vi "Depth and Stainless Correction Pop Up 2016.vi"(6 "New Number\n of Stainless\n(Count)":i32, 7 "Input \nCorrected \nDepth (Feet)":sgl format="%.2f") -> (0 "Array":u16[](array[numeric]), 1 "Record IK Reason 2":bool, 2 "Feet of\nStainless to be\nUsed (Count)":i32, 3 "Depth to \nbe Used \n(Feet)":sgl format="%.2f", 4 "IK Log Note 2":string, 5 "End of Hole 2":u16(ring) items=["ROP Dropped below threshold", "Sudden hard refusal", "Reached target depth", "Broken down hole equipment", "Other"])   [LabVIEW 2016]
doc: "This vi allows the clinician to input the starting flexion. It used in order to derive a flexion correction."
panel:
  in  "End of Hole":u16(ring)=4 items=["ROP Dropped below threshold", "Sudden hard refusal", "Reached target depth", "Broken down hole equipment", "Other"]
  in  "IK Log Note":string
  out "loop counter":i32
  in  "Select Entry \nfor IK Log":u16(ring)=3 items=["IK Increase", "IK stayed the Same", "IK decreased", "Other"]
  in  "Record IK Reason":bool
  out "Original \nUncorrected \nDepth (Feet)":sgl format="%.2f"
  out "Original Feet\n of Stainless\n(Count)":i32
  in  "stop":bool
  in  "Increment Stainless":bool
  in  "Stainless OK As Is":bool
  in  "Correct Stainless":bool
  in  "Depth OK As Is":bool
  in  "Correct Depth":bool
  # "Please Choose \nto Correct Depth\nor to Leave As Is"
  # "Please Choose \nto Correct, Increment, or to \nLeave Feet of Stainless as is"
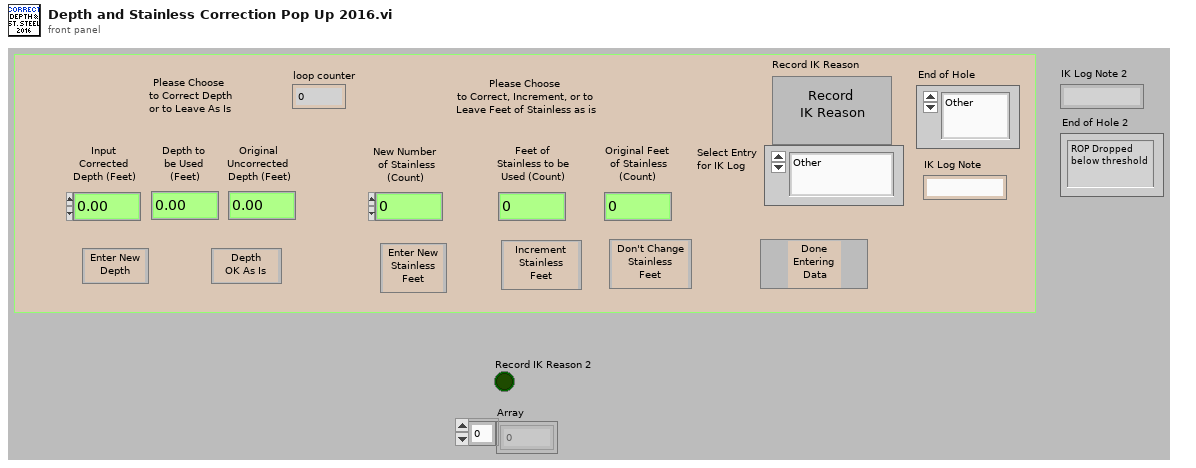
[diagram p1: front panel]
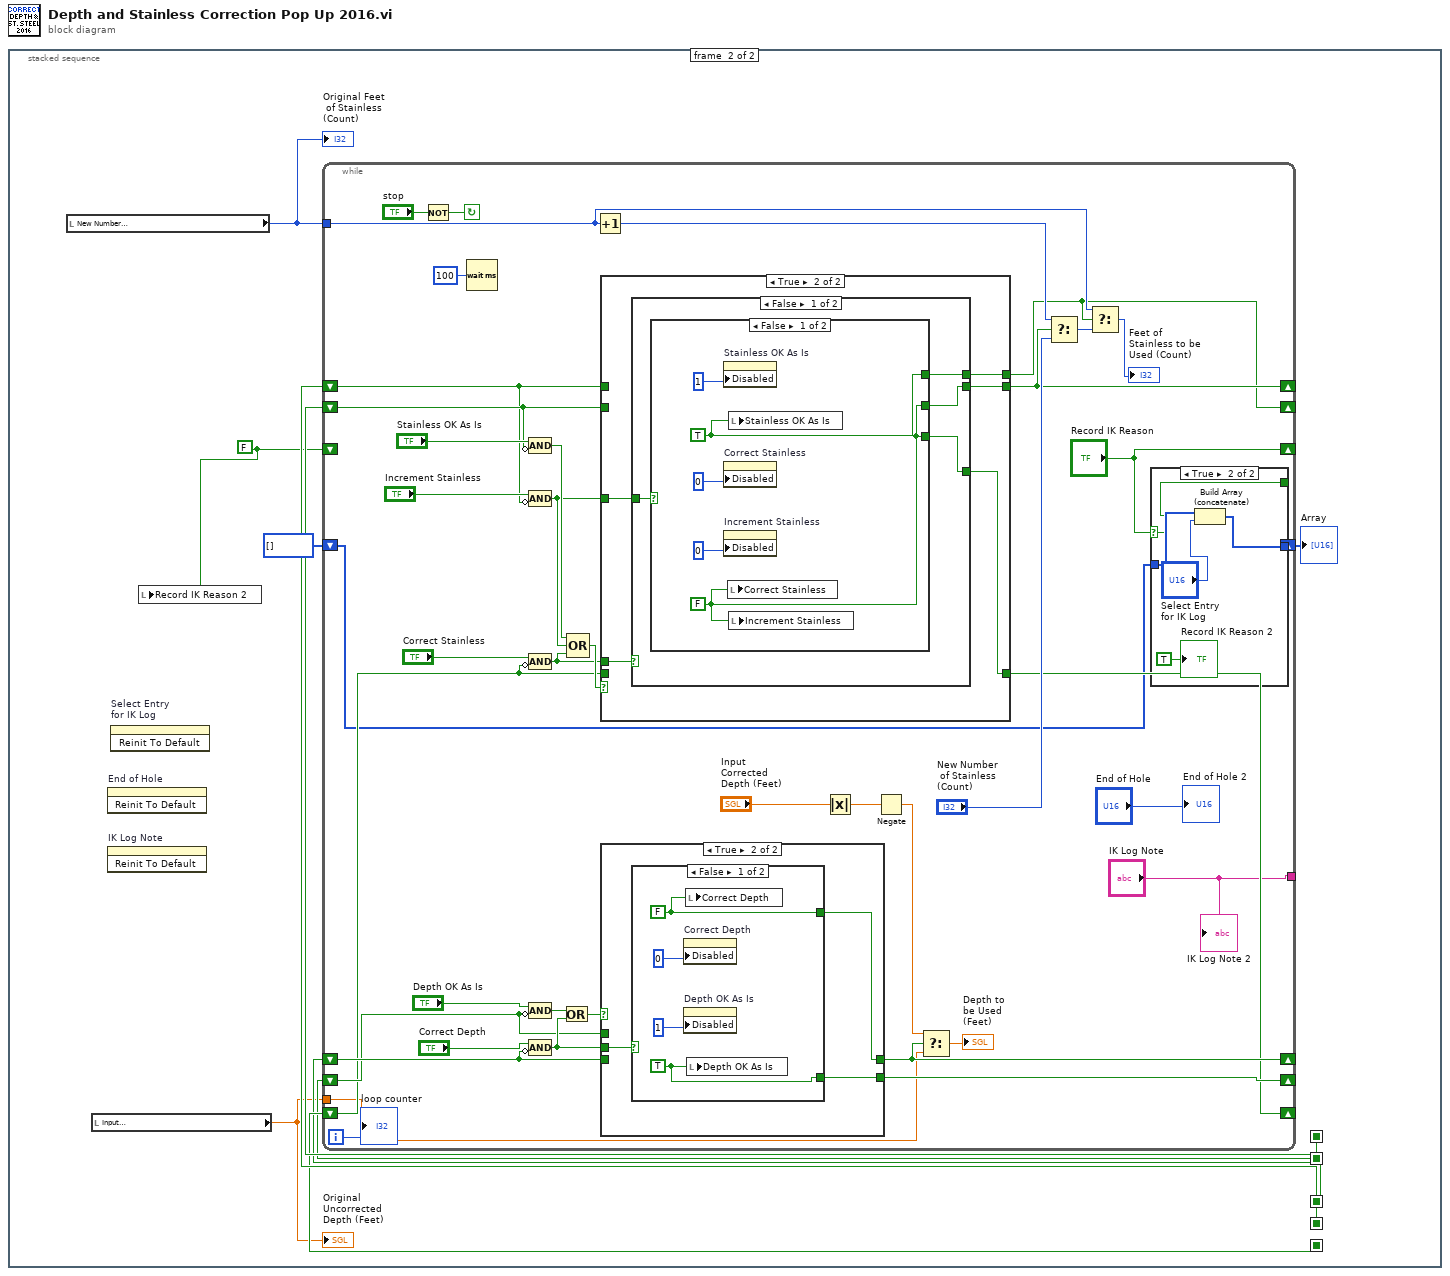
[diagram p0: block diagram]
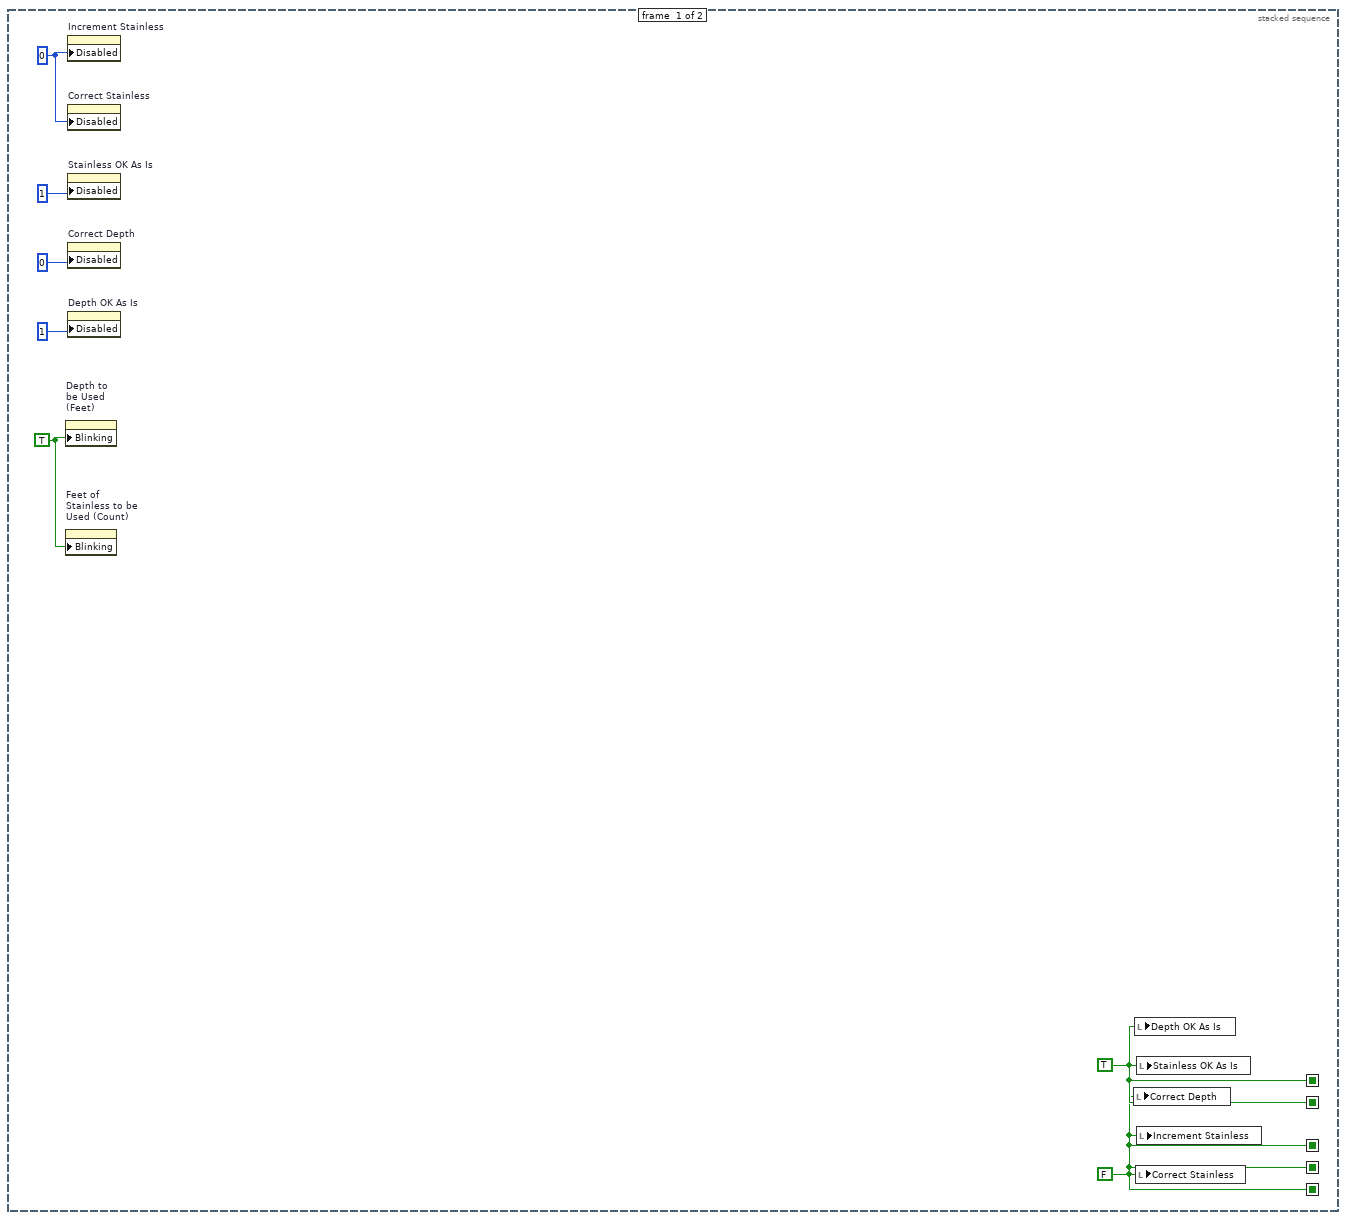
[diagram p2: hidden frame]
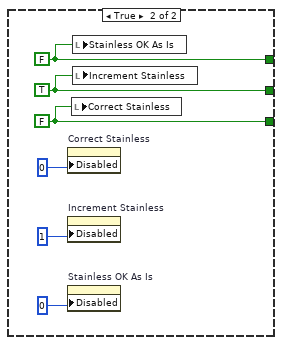
[diagram p5: hidden frame]
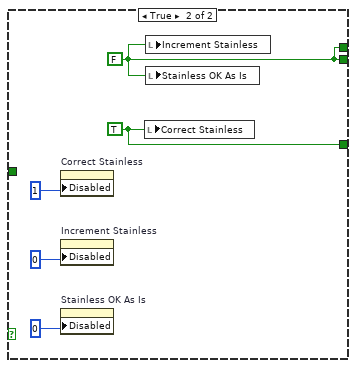
[diagram p6: hidden frame]
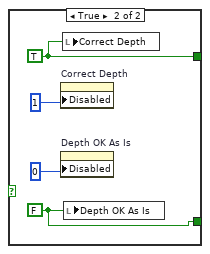
[diagram p8: hidden frame]
diagram:
  n1 = stacked-sequence {
    seq-local: [w6 _] -> [_ w15]
    seq-local: [w6 _] -> [_ w16]
    seq-local: [w7 _] -> [_ w17]
    seq-local: [w6 _] -> [_ w13]
    seq-local: [w7 _] -> [_ w14]
    frame #0 {
      w1 = TRUE
      w2 = 0
      w7 = TRUE
      w6 = FALSE
      n2 = property on="Depth to \nbe Used \n(Feet)" class="DigNum (strict)"("Blinking"=w1) -> ()  [unwired: 2 in, 2 out]
      n3 = property on="Feet of\nStainless to be\nUsed (Count)" class="DigNum (strict)"("Blinking"=w1) -> ()  [unwired: 2 in, 2 out]
      n4 = property on="Increment Stainless" class="Bool (strict)"("Disabled"=w2) -> ()  [unwired: 2 in, 2 out]
      n5 = property on="Correct Stainless" class="Bool (strict)"("Disabled"=w2) -> ()  [unwired: 2 in, 2 out]
      n6 = property on="Stainless OK As Is" class="Bool (strict)"("Disabled"=1) -> ()  [unwired: 2 in, 2 out]
      n7 = property on="Correct Depth" class="Bool (strict)"("Disabled"=0) -> ()  [unwired: 2 in, 2 out]
      n8 = property on="Depth OK As Is" class="Bool (strict)"("Disabled"=1) -> ()  [unwired: 2 in, 2 out]
      n9 = local write "Correct Depth"(w6) -> ()
      n10 = local write "Depth OK As Is"(w7) -> ()
      n11 = local write "Correct Stainless"(w6) -> ()
      n12 = local write "Stainless OK As Is"(w7) -> ()
      n13 = local write "Increment Stainless"(w6) -> ()
    }
    frame #1 {
      w8 = FALSE
      n14 = local read "New Number\n of Stainless\n(Count)"() -> (w12:i32)
      "Original Feet\n of Stainless\n(Count)" <- w12
      n15 = local read "Input \nCorrected \nDepth (Feet)"() -> (w11:sgl)
      "Original \nUncorrected \nDepth (Feet)" <- w11
      n16 = invoke on="End of Hole" class="Ring (strict)" method="Reinit To Default"() -> ()  [unwired: 3 in, 3 out]
      n17 = invoke on="IK Log Note" class="Str" method="Reinit To Default"() -> ()  [unwired: 3 in, 3 out]
      n18 = invoke on="Select Entry \nfor IK Log" class="Ring (strict)" method="Reinit To Default"() -> ()  [unwired: 3 in, 3 out]
      n19 = local write "Record IK Reason 2"(w8) -> ()
      n20 = while {
        tunnel: w11 -> [w29]
        tunnel: w12 -> [w30]
        shift-left: w13 -> [w35]
        shift-right: [w46] -> _
        shift-left: w14 -> [w34]
        shift-right: [w47] -> _
        shift-left: w15 -> [w32]
        shift-right: [w39] -> _
        shift-left: w16 -> [w31]
        shift-right: [w40] -> _
        shift-left: w17 -> [w33]
        shift-right: [w28] -> _
        shift-right: [w24] -> w9
        shift-left: u16[] [] -> [w23]
        shift-right: ["Record IK Reason"] -> _
        shift-left: w8 -> [_]
        tunnel: ["IK Log Note"] -> _
        i -> [w22]
        stop <- w36 continue-if-true
        n21 = Not(x="stop") -> (.not. x?=w36:bool)
        n22 = Wait (ms)(milliseconds to wait=u32 100) -> ()  [unwired: 1 out]
        n23 = Compound Arithmetic op=AND("Stainless OK As Is", invert w33) -> (w42:bool)
        n24 = Compound Arithmetic op=AND("Increment Stainless", invert w31) -> (w37:bool)
        n25 = Compound Arithmetic op=AND("Correct Stainless", invert w32) -> (w38:bool)
        n26 = Compound Arithmetic op=AND("Depth OK As Is", invert w34) -> (w51:bool)
        n27 = Compound Arithmetic op=AND("Correct Depth", invert w35) -> (w49:bool)
        n28 = Or(x=w51, y=w49) -> (x .or. y?=w50:bool)
        n29 = Compound Arithmetic op=OR(w42, w37, w38) -> (w41:bool)
        n30 = Increment(x=w30) -> (x+1=w57:i32)
        n31 = case shown="True" w41 {
          tunnel: [w68 w71] -> w28
          tunnel: [w67 w70] -> w40
          tunnel: [w66 w72] -> w39
          tunnel: w38 -> [_ w73]
          tunnel: w37 -> [_ w69]
          tunnel: w33 -> [w68 _]
          tunnel: w32 -> [w66 _]
          tunnel: w31 -> [w67 _]
          frame False {
          }
          frame True {
            n32 = case shown="False" w73 {
              tunnel: [w74 w93] -> w72
              tunnel: [w76 w92] -> w71
              tunnel: [w75 w92] -> w70
              tunnel: w69 -> [w77 _]
              frame False {
                n33 = case shown="False" w77 {
                  tunnel: [w81 w86] -> w76
                  tunnel: [w82 w87] -> w75
                  tunnel: [w82 w88] -> w74
                  frame False {
                    w81 = TRUE
                    w82 = FALSE
                    n34 = property on="Stainless OK As Is" class="Bool (strict)"("Disabled"=1) -> ()  [unwired: 2 in, 2 out]
                    n35 = property on="Correct Stainless" class="Bool (strict)"("Disabled"=0) -> ()  [unwired: 2 in, 2 out]
                    n36 = property on="Increment Stainless" class="Bool (strict)"("Disabled"=0) -> ()  [unwired: 2 in, 2 out]
                    n37 = local write "Correct Stainless"(w82) -> ()
                    n38 = local write "Stainless OK As Is"(w81) -> ()
                    n39 = local write "Increment Stainless"(w82) -> ()
                  }
                  frame True {
                    w86 = FALSE
                    w87 = TRUE
                    w88 = FALSE
                    n40 = property on="Correct Stainless" class="Bool (strict)"("Disabled"=0) -> ()  [unwired: 2 in, 2 out]
                    n41 = property on="Increment Stainless" class="Bool (strict)"("Disabled"=1) -> ()  [unwired: 2 in, 2 out]
                    n42 = property on="Stainless OK As Is" class="Bool (strict)"("Disabled"=0) -> ()  [unwired: 2 in, 2 out]
                    n43 = local write "Correct Stainless"(w88) -> ()
                    n44 = local write "Stainless OK As Is"(w86) -> ()
                    n45 = local write "Increment Stainless"(w87) -> ()
                  }
                }
              }
              frame True {
                w92 = FALSE
                w93 = TRUE
                n46 = property on="Correct Stainless" class="Bool (strict)"("Disabled"=1) -> ()  [unwired: 2 in, 2 out]
                n47 = property on="Increment Stainless" class="Bool (strict)"("Disabled"=0) -> ()  [unwired: 2 in, 2 out]
                n48 = property on="Stainless OK As Is" class="Bool (strict)"("Disabled"=0) -> ()  [unwired: 2 in, 2 out]
                n49 = local write "Correct Stainless"(w93) -> ()
                n50 = local write "Increment Stainless"(w92) -> ()
                n51 = local write "Stainless OK As Is"(w92) -> ()
              }
            }
          }
        }
        n52 = case shown="True" w50 {
          tunnel: w49 -> [_ w98]
          tunnel: [w95 w96] -> w47
          tunnel: [w94 w97] -> w46
          tunnel: w35 -> [w94 _]
          tunnel: w34 -> [w95 _]
          frame False {
          }
          frame True {
            n53 = case shown="False" w98 {
              tunnel: [w102 w106] -> w97
              tunnel: [w101 w105] -> w96
              frame False {
                w102 = FALSE
                w101 = TRUE
                n54 = property on="Correct Depth" class="Bool (strict)"("Disabled"=0) -> ()  [unwired: 2 in, 2 out]
                n55 = property on="Depth OK As Is" class="Bool (strict)"("Disabled"=1) -> ()  [unwired: 2 in, 2 out]
                n56 = local write "Correct Depth"(w102) -> ()
                n57 = local write "Depth OK As Is"(w101) -> ()
              }
              frame True {
                w105 = FALSE
                w106 = TRUE
                n58 = property on="Correct Depth" class="Bool (strict)"("Disabled"=1) -> ()  [unwired: 2 in, 2 out]
                n59 = property on="Depth OK As Is" class="Bool (strict)"("Disabled"=0) -> ()  [unwired: 2 in, 2 out]
                n60 = local write "Correct Depth"(w106) -> ()
                n61 = local write "Depth OK As Is"(w105) -> ()
              }
            }
          }
        }
        n62 = Absolute Value(x="Input \nCorrected \nDepth (Feet)") -> (abs(x)=w26:sgl)
        n63 = Negate(x=w26) -> (-x=w25:sgl)
        n64 = Select(t=w25, s=w46, f=w29) -> (s? t:f=→"Depth to \nbe Used \n(Feet)":sgl)
        n65 = Select(t=w57, s=w40, f="New Number\n of Stainless\n(Count)") -> (s? t:f=w56:i32)
        n66 = Select(t=w30, s=w28, f=w56) -> (s? t:f=→"Feet of\nStainless to be\nUsed (Count)":i32)
        n67 = case shown="True" "Record IK Reason" {
          selector: "Record IK Reason" -> [w59 w62]
          tunnel: [w60 w64] -> w24
          tunnel: w23 -> [w60 w65]
          tunnel: [w59 w62] -> _
          frame False {
          }
          frame True {
            n68 = Build Array (concatenate)(w65, "Select Entry \nfor IK Log") -> (w64:u16[])
            "Record IK Reason 2" <- TRUE ("Record IK Reason 2")
          }
        }
        "loop counter" <- w22
        "IK Log Note 2" <- "IK Log Note"
        "End of Hole 2" <- "End of Hole"
      }
      "Array" <- w9
    }
  }
